vi "Read.vi"(11 "PathValue in":refnum<class "PathValue.lvclass">) -> (2 "Path":path)   [LabVIEW 2020, in "Volatus.lvlib" / "PathValue.lvclass"]
uses:
  PathValue.lvclass
  PathValue.lvclass/PathValue.ctl
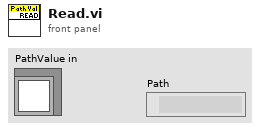
[diagram p1: front panel]
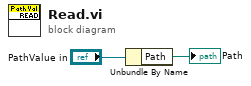
[diagram p0: block diagram]
diagram:
  n1 = Unbundle By Name("PathValue in") -> ("Path"=→"Path":path)
